vi "GetMagnitude.vi"(8 "error in (no error)":errorcluster, 11 "LIA in":refnum<class "LIA.lvclass">) -> (0 "error out":errorcluster, 2 "Magnitude":dbl, 3 "LIA out":refnum<class "LIA.lvclass">)   [LabVIEW 2017, in "LIA.lvclass"]
uses:
  LIA.lvclass
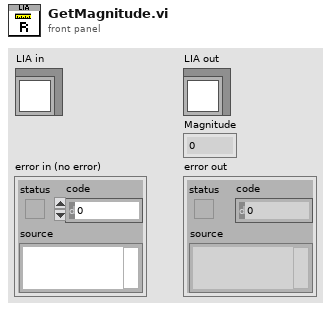
[diagram p1: front panel]
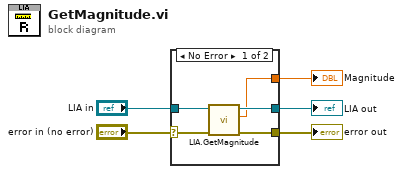
[diagram p0: block diagram]
diagram:
  n1 = case shown="No Error" "error in (no error)" {
    selector: "error in (no error)" -> [w8 w12]
    tunnel: [w7 w12] -> w4
    tunnel: [w9 w11] -> w2
    tunnel: "LIA in" -> [w10 w11]
    tunnel: [w6 _] -> w1
    frame No Error {
      n2 = call-dynamic "LIA.GetMagnitude.vi"("error in (no error)"=w8, "LIA in"=w10) -> ("error out"=w7:errorcluster, "Magnitude"=w6:dbl, "LIA out"=w9:refnum<class "LIA.lvclass">)  [unwired: 7 in]
    }
    frame Error {
    }
  }
  "error out" <- w4
  "LIA out" <- w2
  "Magnitude" <- w1
